vi "PXIe-7902 Getting Started feat Frequency Shift (FPGA).vi"() -> ()   [LabVIEW 2024]
doc: "Controls the generation and reception of data transferred from the Host to the FPGA.\nPort 0 receives data from the Port 0 TX Input DMA FIFO and transmits that data to Port 1.\nPort 1 receives data from the Port 1 TX Input DMA FIFO and transmits that data to Port 0."
uses:
  <instrlib>/_niInstr/Streaming/v1/Common/Stream State.ctl
  <instrlib>/FlexRIO/DRAM FIFO/v2/FPGA/DRAM FIFO/DRAM FIFO Status.ctl
  Controls/Data Paths.ctl
  Controls/Data Triggers.ctl
  <vilib>/Platform/TimedLoop/XDataNode/timing_clust.ctl
  <vilib>/Platform/TimedLoop/XDataNode/nitl_modes.ctl
  <vilib>/Platform/TimedLoop/XDataNode/wakeup.ctl
  <instrlib>/FlexRIO/DRAM FIFO/v2/FPGA/DRAM FIFO/FIFO Depth.ctl
  <vilib>/rvi/Emulation/niFpgaSctlEmulationGetInTimedLoop.vi
  <vilib>/rvi/Emulation/niFpgaEmulationReportErrorSimple.vi
  <vilib>/rvi/Emulation/niFpgaGetClockAttributes.vi
  <vilib>/rvi/Emulation/niFpgaCriticalErrorInLSC.vi
  <vilib>/rvi/interface/RandomDataEmulation/nirviRandomDataMultiElementFPGAFIFO.vi
  <instcachedir>/0/nirviRandomDataMultiElementFPGAFIFO_BE2FF10D3D6E420AB0291A02835C249E.lvgen/nirviRandomDataMultiElementFPGAFIFO_BE2FF10D3D6E420AB0291A02835C249E_000.vi
  <vilib>/rvi/interface/RandomDataEmulation/niFpgaRandomDataHandleErrors.vi
  <vilib>/Platform/TimedLoop/XDataNode/XDataNode.xnode
  <vilib>/rvi/DataTransferAndStorage/Container/XNode/niFpgaContainer.xnode
  <vilib>/rvi/interface/RandomDataEmulation/nirviRandomDataFpgaMultiElementTemplate.vi
  <vilib>/rvi/FIFO/Fifo_Resource/nirvififoEmulationP2P.vi
  <instrlib>/FlexRIO/DRAM FIFO/v2/FPGA/DRAM FIFO/Unpack U16.vi
  <instrlib>/FlexRIO/DRAM FIFO/v2/FPGA/DRAM FIFO/Pack U16.vi
  <instrlib>/FlexRIO/DRAM FIFO/v2/FPGA/DRAM FIFO/Private/DRAM FIFO U512/Create 512x1 DRAM FIFO.vi
  <vilib>/Platform/TimedLoop/XDataNode/XDNodeRunTimeDep.lvlib
  <instrlib>/_niInstr/Streaming/v1/FPGA/niInstr Streaming v1 FPGA.lvlib
  <instrlib>/_niInstr/Streaming/v1/Common/niInstr Streaming v1 Common.lvlib
  <instrlib>/FlexRIO/DRAM FIFO/v2/FPGA/DRAM FIFO/DRAM FIFO v2 FPGA.lvclass
  <instrlib>/_niInstr/DSP/v1/FPGA/niInstr DSP v1 FPGA.lvlib
  <instrlib>/FlexRIO/DRAM FIFO/v2/FPGA/DRAM FIFO/Private/DRAM FIFO U512/DRAM FIFO U512 v2 FPGA.lvclass
  <instrlib>/_niInstr/DSP/v1/FPGA/Public/Sub VIs/Data Conversion/IQ to I16 - N spc - S18.1.vi
  <instrlib>/_niInstr/DSP/v1/FPGA/Public/Sub VIs/Data Conversion/I16 to IQ - N spc - S18.1.vi
  <instrlib>/_niInstr/DSP/v1/FPGA/Public/Sub VIs/Frequency Shift/Frequency Shift - 8 spc.vi
panel:
  in  "Tab Control":T1(tab)=enum."DRAM FIFO"
  in  "stream.request state 0":T2
  in  "stream.num samples 0":u64
  out "stream.metadata 0":u64
  out "stream.samples transferred 0":u64
  out "stream.state 0":T2
  in  "Data Source":T3
  in  "Data Sink":T3
  in  "Data Source Trigger":T4
  in  "SW Trigger":bool
  out "DRAM FIFO Status":T5
  in  "read grant time":u16=100
  in  "write grant time":u16=100
  in  "frequency shift":fxp<+/-,48,0>
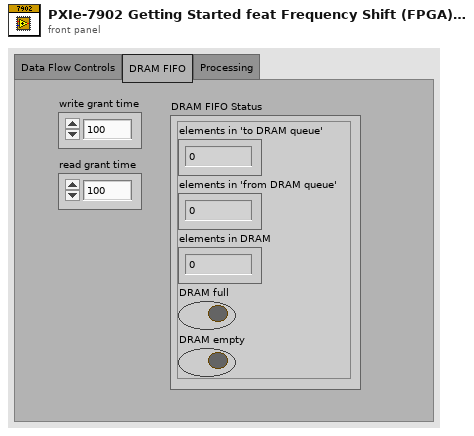
[diagram p1: front panel]
types:
  T1 = enum32{"Data Flow Controls", "DRAM FIFO", "Processing"}
  T2 = typedef "niInstr Streaming v1 Common.lvlib/Stream State.ctl" = enum8{"Idle", "Finite Transfer", "Continuous", "Done", "Error", "Not Ready", "Cancel"}
  T3 = typedef "Data Paths.ctl" = enum16{"DMA", "P2P"}
  T4 = typedef "Data Triggers.ctl" = enum16{"Valid Data", "Software"}
  T5 = typedef "DRAM FIFO v2 FPGA.lvclass/DRAM FIFO Status.ctl" = cluster{"elements in 'to DRAM queue'":u32, "elements in 'from DRAM queue'":u32, "elements in DRAM":u32, "DRAM full":bool, "DRAM empty":bool}
  T6 = typedef "DRAM FIFO v2 FPGA.lvclass/FIFO Depth.ctl" = u8
  T7 = typedef "XDNodeRunTimeDep.lvlib/timing_clust.ctl" = cluster{"Expected End [f-1]":u64, "Actual End [f-1]":u64, "Finished Late? [f-1]":bool, "Expected End [i-1]":u64, "Actual End [i-1]":u64, "Finished Late? [i-1]":bool, "Expected Start [i]":u64, "Actual Start [i]":u64, "Expected Start [f]":u64, "Actual Start [f]":u64, "Source Name":string, "Structure Name":string, "Period":i64, "Deadline":i64, "Offset":i64, "Start":i64, "Priority":i32, "Timeout":i32, "Mode":T8, "Wakeup Reason":T9, "Error":errorcluster, "Source Type":string, "Secondary Source Type":string, "Global End Time":u64, "Global Start Time":u64, "Frame Duration":u64, "Iteration Duration":u64, "Assigned CPU":i32, "I/O Scan Engine Mode":u32}
  T8 = typedef "XDNodeRunTimeDep.lvlib/nitl_modes.ctl" = enum32{"No Change", "Process missed periods, maintain original phase", "Discard missed periods, maintain original phase", "Process missed periods, ignore original phase", "Discard missed periods, ignore original phase"}
  T9 = typedef "XDNodeRunTimeDep.lvlib/wakeup.ctl" = enum32{"Normal", "Aborted", "Asynchronous wakeup", "Timing source error", "Timed loop error", "Timeout"}
  T10 = typedef "niInstr DSP v1 Shared.lvlib/IQ Data.ctl" = cluster{"I":fxp<+/-,18,1>, "Q":fxp<+/-,18,1>, "overflow":bool}
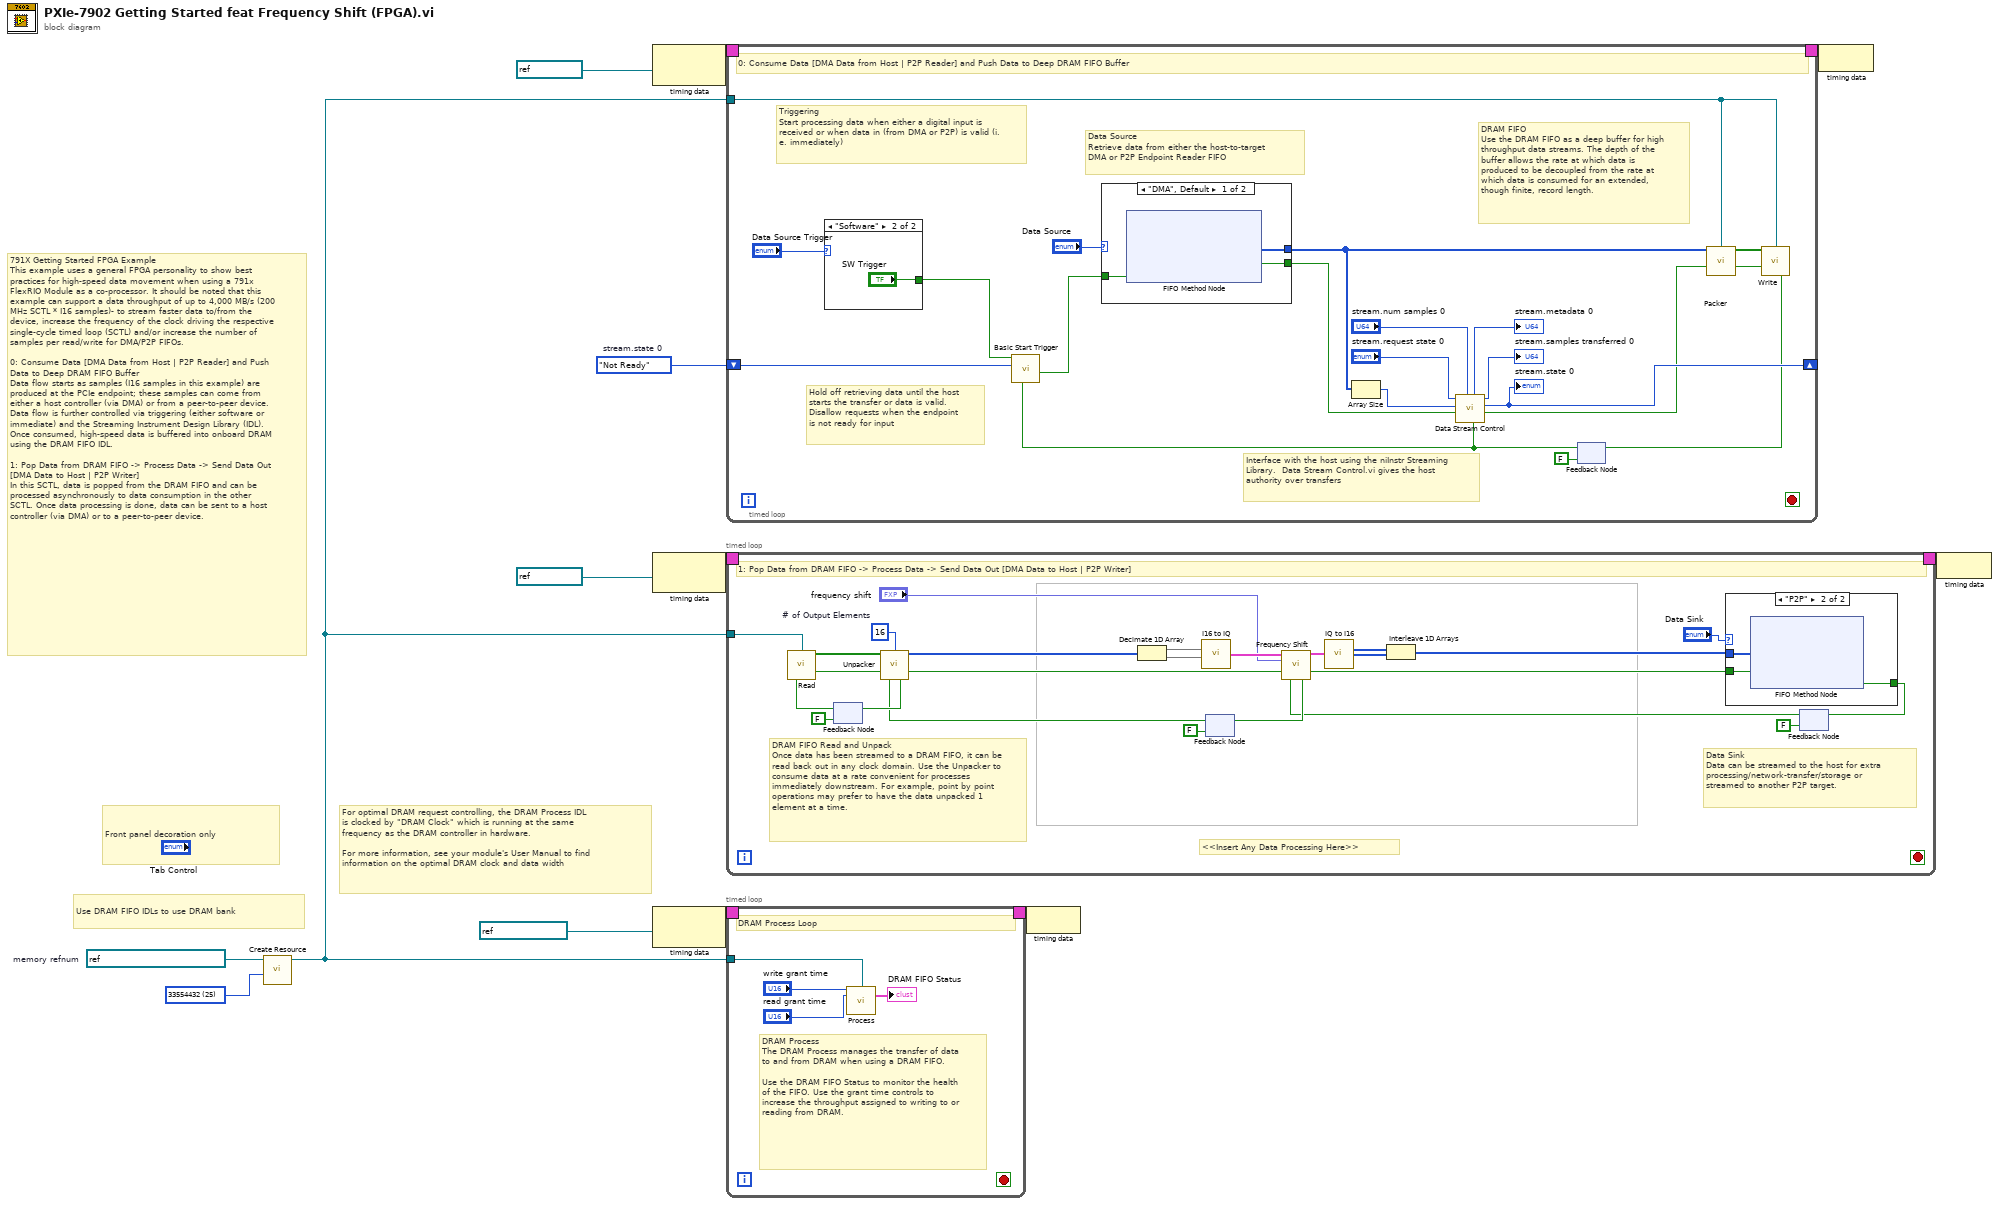
[diagram p0: block diagram]
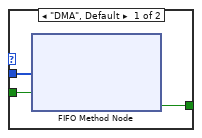
[diagram p2: hidden frame]
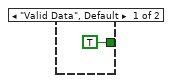
[diagram p3: hidden frame]
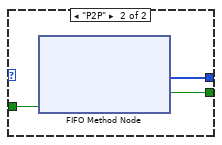
[diagram p4: hidden frame]
diagram:
  w1 = refnum<k21> "DRAM_FIFO0_33554432"  # memory refnum
  w3 = T6 25 items=["4"=2, "8"=3, "16"=4, "32"=5, "64"=6, "128"=7, "256"=8, "512"=9, "1024"=10, "2048"=11, "4096"=12, "8192"=13, "16384"=14, "32768"=15, "65536"=16, "131072"=17, "262144"=18, "524288"=19, "1048576"=20, "2097152"=21, "4194304"=22, "8388608"=23, "16777216"=24, "33554432"=25, "67108864"=26, "134217728"=27, "268435456"=28, "536870912"=29, "1073741824"=30, "2147483648"=31, "4294967296"=32] ("actual # of DRAM elements")
  w10 = Stream_State."Not Ready"  # stream.state 0
  # "791X Getting Started FPGA Example\nThis example uses a general FPGA personality to show best practices for high-speed data movement when using a 791x FlexRIO Module as a co-processor. It should be noted that this example can support a data throughput of up to 4,000 MB/s (200 MHz SCTL * I16 samples)- to stream faster data to/from the device, increase the frequency of the clock driving the respective single-cycle timed loop (SCTL) and/or increase the number of samples per read/write for DMA/P2P FIFOs.\n\n0: Consume Data [DMA Data from Host | P2P Reader] and Push Data to Deep DRAM FIFO Buffer\nData flow starts as samples (I16 samples in this example) are produced at the PCIe endpoint; these samples can come from either a host controller (via DMA) or from a peer-to-peer device. Data flow is further controlled via triggering (either software or immediate) and the Streaming Instrument Design Library (IDL). Once consumed, high-speed data is buffered into onboard DRAM using the DRAM FIFO IDL.\n\n1: Pop Data from DRAM FIFO -> Process Data -> Send Data Out [DMA Data to Host | P2P Writer]\nIn this SCTL, data is popped from the DRAM FIFO and can be processed asynchronously to data consumption in the other SCTL. Once data processing is done, data can be sent to a host controller (via DMA) or to a peer-to-peer device."
  # "For optimal DRAM request controlling, the DRAM Process IDL\nis clocked by \"DRAM Clock\" which is running at the same \nfrequency as the DRAM controller in hardware.\n\nFor more information, see your module's User Manual to find\ninformation on the optimal DRAM clock and data width"
  # "Use DRAM FIFO IDLs to use DRAM bank"
  # "Front panel decoration only"
  n1 = call-poly <instrlib>:"Create Resource.vi"("actual # of DRAM elements"=w3, "memory refnum"=w1) -> ("DRAM FIFO ref out"=w2:refnum<class "DRAM FIFO v2 FPGA.lvclass">)  [unwired: 9 in]
  n2 = node-c288(refnum<k21> "200MHz" ("Source Name")) -> (w13:T7)
  n3 = node-c288(refnum<k21> "200MHz" ("Source Name")) -> (w6:T7)
  n4 = node-c288(refnum<k21> "DRAM Clock" ("Source Name")) -> (w9:T7)
  n5 = timed-loop {
    timing: w13 -> [_]
    timing-out: [_] -> w12
    shift-right: [w33] -> _
    shift-left: w10 -> [w28]
    tunnel: w2 -> [w14]
    stop <- _ stop-if-true
    # "DRAM FIFO  \nUse the DRAM FIFO as a deep buffer for high throughput data streams. The depth of the buffer allows the rate at which data is produced to be decoupled from the rate at which data is consumed for an extended, though finite, record length."
    # "Triggering\nStart processing data when either a digital input is received or when data in (from DMA or P2P) is valid (i.e. immediately)"
    # "Data Source\nRetrieve data from either the host-to-target DMA or P2P Endpoint Reader FIFO"
    # "Interface with the host using the niInstr Streaming Library.  Data Stream Control.vi gives the host authority over transfers"
    # "Hold off retrieving data until the host starts the transfer or data is valid.  Disallow requests when the endpoint is not ready for input"
    # "0: Consume Data [DMA Data from Host | P2P Reader] and Push Data to Deep DRAM FIFO Buffer"
    n6 = case shown="\"Software\"" "Data Source Trigger" {
      tunnel: [TRUE "SW Trigger"] -> w22
      frame "Valid Data", Default {
      }
      frame "Software" {
      }
    }
    n7 = feedback #1(FALSE ("ready for input")) -> (w17:bool)
    n8 = call <instrlib>:"Basic Start Trigger.vi"("ready for start trigger"=w17, "stream.state"=w28, "start trigger"=w22) -> ("data valid"=w18:bool)  [unwired: 8 in]
    n9 = case shown="\"DMA\", Default" "Data Source" {
      tunnel: [w38 w41] -> w21
      tunnel: [w37 w39] -> w25
      tunnel: w18 -> [w36 w40]
      frame "DMA", Default {
        n10 = xnode ("FIFO Method Node")("Ready for Output"=w36) -> ("Element"=w38:i16[], "Output Valid"=w37:bool)  [unwired: 1 in, 1 out]
      }
      frame "P2P" {
        n11 = xnode ("FIFO Method Node")("Ready for Output"=w40) -> ("Element"=w41:i16[], "Output Valid"=w39:bool)  [unwired: 1 in, 1 out]
      }
    }
    n12 = Array Size(array=w21) -> (size(s)=w27:i32)
    n13 = call <instrlib>:"Data Stream Control.vi"("ready for input?"=w17, "stream.num samples 0"="stream.num samples 0", "data valid"=w25, "element count"=w27, "stream.request state 0"="stream.request state 0") -> ("send data"=w20:bool, "stream.state 0"=w33:T2, "stream.samples transferred 0"=→"stream.samples transferred 0":u64, "stream.metadata 0"=→"stream.metadata 0":u64)  [unwired: 2 in, 1 out]
    "stream.state 0" <- w33
    n14 = call-poly <instrlib>:"Packer.vi"("data in"=w21, "DRAM FIFO in"=w14, "input valid"=w20) -> ("data out"=w19:bool[], "output valid"=w15:bool)  [unwired: 10 in, 1 out]
    n15 = call <instrlib>:"Write.vi"("element"=w19, "DRAM FIFO ref in"=w14, "input valid"=w15) -> ("ready for input"=w16:bool)  [unwired: 12 in]
    n16 = feedback-in #1(w16) -> ()
  }
  n17 = timed-loop {
    timing: w6 -> [_]
    timing-out: [_] -> w5
    tunnel: w2 -> [w68]
    stop <- _ stop-if-true
    w60 = u16 16  # # of Output Elements
    # "<<Insert Any Data Processing Here>>"
    # "Data Sink\nData can be streamed to the host for extra processing/network-transfer/storage or streamed to another P2P target."
    # "DRAM FIFO Read and Unpack\nOnce data has been streamed to a DRAM FIFO, it can be read back out in any clock domain. Use the Unpacker to consume data at a rate convenient for processes immediately downstream. For example, point by point operations may prefer to have the data unpacked 1 element at a time."
    # "1: Pop Data from DRAM FIFO -> Process Data -> Send Data Out [DMA Data to Host | P2P Writer]"
    n18 = feedback #2(FALSE ("ready for input")) -> (w64:bool)
    n19 = call <instrlib>:"Read.vi"("DRAM FIFO ref in"=w68, "ready for output"=w64) -> ("element"=w67:bool[], "output valid"=w66:bool)  [unwired: 12 in]
    n20 = feedback #3(FALSE ("ready for input")) -> (w54:bool)
    n21 = call-poly <instrlib>:"Unpacker.vi"("packed data in"=w67, "output data size (elements)"=w60, "input valid"=w66, "ready for output"=w54) -> ("unpacked data out"=w47:u16[], "output valid"=w58:bool, "ready for input"=w65:bool)  [unwired: 9 in]
    n22 = feedback-in #2(w65) -> ()
    n23 = Decimate 1D Array(w47) -> (w46:u16[], w45:u16[])
    n24 = call-poly <instrlib>:"I16 to IQ.vi"("I"=w46, "Q"=w45) -> ("IQ"=w52:T10[])  [unwired: 13 in]
    n25 = feedback #4(FALSE ("Ready for Input")) -> (w53:bool)
    n26 = call-poly <instrlib>:"Frequency Shift.vi"("data in"=w52, "frequency shift"="frequency shift", "input valid"=w58, "ready for output (T)"=w53) -> ("data out"=w51:T10[], "output valid"=w57:bool, "ready for input"=w55:bool)  [unwired: 8 in, 1 out]
    n27 = feedback-in #3(w55) -> ()
    n28 = call-poly <instrlib>:"IQ to I16.vi"("IQ"=w51) -> ("I"=w50:i16[], "Q"=w49:i16[])  [unwired: 12 in, 1 out]
    n29 = Interleave 1D Arrays(w50, w49) -> (w48:i16[])
    n30 = case shown="\"P2P\"" "Data Sink" {
      tunnel: [w71 w72] -> w63
      tunnel: w48 -> [w70 w74]
      tunnel: w57 -> [w69 w73]
      frame "DMA", Default {
        n31 = xnode ("FIFO Method Node")("Element"=w70, "Input Valid"=w69) -> ("Ready for Input"=w71:bool)  [unwired: 1 in, 1 out]
      }
      frame "P2P" {
        n32 = xnode ("FIFO Method Node")("Element"=w74, "Input Valid"=w73) -> ("Ready for Input"=w72:bool)  [unwired: 1 in, 1 out]
      }
    }
    n33 = feedback-in #4(w63) -> ()
  }
  n34 = timed-loop {
    timing: w9 -> [_]
    timing-out: [_] -> w8
    tunnel: w2 -> [w80]
    stop <- _ stop-if-true
    # "DRAM Process\nThe DRAM Process manages the transfer of data to and from DRAM when using a DRAM FIFO. \n\nUse the DRAM FIFO Status to monitor the health of the FIFO. Use the grant time controls to increase the throughput assigned to writing to or reading from DRAM."
    # "DRAM Process Loop"
    n35 = call <instrlib>:"Process.vi"("write grant time (clock ticks)"="write grant time", "DRAM FIFO ref in"=w80, "read grant time (clock ticks)"="read grant time") -> ("status"=→"DRAM FIFO Status":T5)  [unwired: 11 in, 1 out]
  }
  n36 = node-c288(w8) -> ()
  n37 = node-c288(w12) -> ()
  n38 = node-c288(w5) -> ()
